vi "Check Aurora Link.vi"(0 "niUsrpRio Session":T2={"FPGA Interface"=refnum, "RIO Interface Number"=0, "Data Clock Rate"=0, "FPGA Data Clock Rate"=0, "Global Settings Register Bus"=refnum, "Radio 0 Settings Register Bus"=refnum, "Radio 1 Settings Register Bus"=refnum, "Radio Settings Bus Semaphore"=refnum, "DB Queues"=[], "Characterization Data Valid?"=FALSE, "EEPROM Header"={"Checksum"=0, "Product Code"=0, "Hardware Current Version"=0, "Hardware Oldest Compatible Version"=0, "EEPROM Map Current Version"=0, "EEPROM Map Oldest Compatible Version"=0, "User Password"="", "Pointer to Factory Header"=0, "Pointer to User Header"=0, "Recommended Interval"=0, "Number of Reserved Bytes"=9, "Number of Daughterboards"=0, "Daughterboard IDs"=[], "Daughterboard Serial Numbers"=[]}, "Device Data Header"={"Checksum"=0, "Number of Channels"=0, "Number of Gain Settings"=[], "Pointer to Characterization Data"=[], "Number of Reserved Bytes"=27, "Number of Frequencies"=[]}, "EEPROM Characterization Header"={"Checksum"=0, "Date"=timestamp(0 s since 1904-01-01), "Temperature"=0.0, "Misc. Info"="", "Pointer to Device Data Header"=0, "Number of Reserved Bytes"=28}, "Characterization Data"=[], "FPGA Current Version"=0, "FPGA Oldest Compatible Version"=0, "Fixed Logic Current Version"=0, "Fixed Logic Oldest Compatible Version"=0, "FPGA Radio Settings Bus Current Version"=0, "FPGA Radio Settings Bus Oldest Compatible Version"=0, "FPGA Board Config Current Version"=0, "FPGA Board Config Oldest Compatible Version"=0, "Daughterboard Clock Rate"=0, "daughterboard configuration session handles"=[]} {"Daughterboard Clock Rate" format="%#.3pHz"; "FPGA Data Clock Rate" format="%#.3pHz"; "Data Clock Rate" format="%#.3pHz"; "Characterization Data"."Frequencies [Hz]" format="%#_6p"; "EEPROM Characterization Header"."Pointer to Device Data Header" format="%x"; "EEPROM Characterization Header"."Checksum" format="%x"; "Device Data Header"."Pointer to Characterization Data" format="%x"; "Device Data Header"."Checksum" format="%x"; "EEPROM Header"."Pointer to User Header" format="%x"; "EEPROM Header"."Pointer to Factory Header" format="%x"; "EEPROM Header"."Product Code" format="%x"; "EEPROM Header"."Checksum" format="%x"}, 11 "error in":errorcluster) -> (4 "niUsrpRio Session (out)":T2={"FPGA Interface"=refnum, "RIO Interface Number"=0, "Data Clock Rate"=0, "FPGA Data Clock Rate"=0, "Global Settings Register Bus"=refnum, "Radio 0 Settings Register Bus"=refnum, "Radio 1 Settings Register Bus"=refnum, "Radio Settings Bus Semaphore"=refnum, "DB Queues"=[], "Characterization Data Valid?"=FALSE, "EEPROM Header"={"Checksum"=0, "Product Code"=0, "Hardware Current Version"=0, "Hardware Oldest Compatible Version"=0, "EEPROM Map Current Version"=0, "EEPROM Map Oldest Compatible Version"=0, "User Password"="", "Pointer to Factory Header"=0, "Pointer to User Header"=0, "Recommended Interval"=0, "Number of Reserved Bytes"=9, "Number of Daughterboards"=0, "Daughterboard IDs"=[], "Daughterboard Serial Numbers"=[]}, "Device Data Header"={"Checksum"=0, "Number of Channels"=0, "Number of Gain Settings"=[], "Pointer to Characterization Data"=[], "Number of Reserved Bytes"=27, "Number of Frequencies"=[]}, "EEPROM Characterization Header"={"Checksum"=0, "Date"=timestamp(0 s since 1904-01-01), "Temperature"=0.0, "Misc. Info"="", "Pointer to Device Data Header"=0, "Number of Reserved Bytes"=28}, "Characterization Data"=[], "FPGA Current Version"=0, "FPGA Oldest Compatible Version"=0, "Fixed Logic Current Version"=0, "Fixed Logic Oldest Compatible Version"=0, "FPGA Radio Settings Bus Current Version"=0, "FPGA Radio Settings Bus Oldest Compatible Version"=0, "FPGA Board Config Current Version"=0, "FPGA Board Config Oldest Compatible Version"=0, "Daughterboard Clock Rate"=0, "daughterboard configuration session handles"=[]} {"Daughterboard Clock Rate" format="%#.3pHz"; "FPGA Data Clock Rate" format="%#.3pHz"; "Data Clock Rate" format="%#.3pHz"; "Characterization Data"."Frequencies [Hz]" format="%#_6p"; "EEPROM Characterization Header"."Pointer to Device Data Header" format="%x"; "EEPROM Characterization Header"."Checksum" format="%x"; "Device Data Header"."Pointer to Characterization Data" format="%x"; "Device Data Header"."Checksum" format="%x"; "EEPROM Header"."Pointer to User Header" format="%x"; "EEPROM Header"."Pointer to Factory Header" format="%x"; "EEPROM Header"."Product Code" format="%x"; "EEPROM Header"."Checksum" format="%x"}, 6 "SFP Port Debug":T1(array[cluster]), 15 "error out":errorcluster)   [LabVIEW 2016]
uses:
  <instrlib>/niUsrpRio/Config/v1/Host/Public/niUsrpRio Session.ctl
  <instrlib>/_niInstr/Register Bus/v0/Host/Public/Register Bus Session.ctl
  <instrlib>/_niInstr/Register Bus/v0/Host/Private/Session Data.ctl
  <instrlib>/niUsrpRio/Config/v1/Host/Private/DB Queue Reference.ctl
  <instrlib>/niUsrpRio/Config/v1/Host/Private/Daughterboard Data.ctl
  <instrlib>/niUsrpRio/Config/v1/Host/Private/ATR state data.ctl
  <instrlib>/niUsrpRio/Config/v1/Host/Private/Antenna Configuration.ctl
  <instrlib>/niUsrpRio/Config/v1/Host/Private/CPLD Power Mode.ctl
  <instrlib>/niUsrpRio/Config/v1/Host/Public/EEPROM Header.ctl
  <instrlib>/niUsrpRio/Config/v1/Host/Public/EEPROM Device Data Header.ctl
  <instrlib>/niUsrpRio/Config/v1/Host/Public/EEPROM Characterization Header.ctl
  <instrlib>/niUsrpRio/Config/v1/Host/Public/Characterization Data.ctl
  <instrlib>/niUsrpRio/Config/v1/Host/Public/IQ Imbalance.ctl
  Aurora FPGA Ref.ctl
  <vilib>/rvi/errors/niLvFpgaAdjustHostInterfaceError.vi
  <vilib>/rvi/interface/nirviReadWriteControl/nirviReadWriteControl.xnode
  <vilib>/rvi/interface/Simulation/niFpgaSimulationCallBeginRW.vi
  NiFpgaLv.dll
  <instrlib>/_niInstr/Register Bus/v0/Host/niInstr Register Bus v0 Host.lvlib
  <instrlib>/niUsrpRio/Config/v1/Host/niUsrpRio Config v1 Host.lvlib
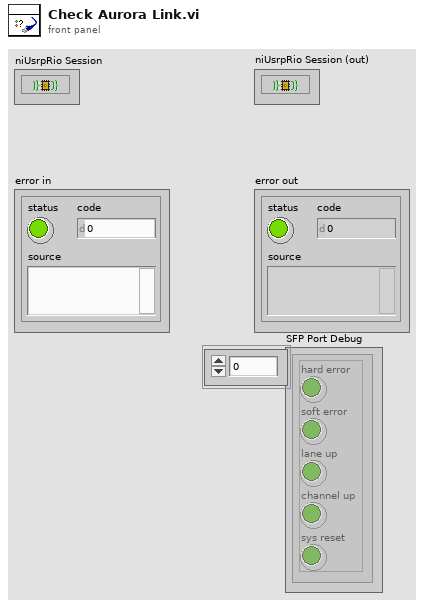
[diagram p1: front panel]
types:
  T1 = cluster{"hard error":bool, "soft error":bool, "lane up":bool, "channel up":bool, "sys reset":bool}[]
  T2 = typedef "niUsrpRio Config v1 Host.lvlib/niUsrpRio Session.ctl" = cluster{"FPGA Interface":refnum<k20>, "RIO Interface Number":u32, "Data Clock Rate":u32, "FPGA Data Clock Rate":u32, "Global Settings Register Bus":T3, "Radio 0 Settings Register Bus":T3, "Radio 1 Settings Register Bus":T3, "Radio Settings Bus Semaphore":T4, "DB Queues":T5[], "Characterization Data Valid?":bool, "EEPROM Header":T6, "Device Data Header":T7, "EEPROM Characterization Header":T8, "Characterization Data":T9[], "FPGA Current Version":u32, "FPGA Oldest Compatible Version":u32, "Fixed Logic Current Version":u32, "Fixed Logic Oldest Compatible Version":u32, "FPGA Radio Settings Bus Current Version":u32, "FPGA Radio Settings Bus Oldest Compatible Version":u32, "FPGA Board Config Current Version":u32, "FPGA Board Config Oldest Compatible Version":u32, "Daughterboard Clock Rate":u32, "daughterboard configuration session handles":u64[]}
  T3 = typedef "niInstr Register Bus v0 Host.lvlib/Register Bus Session.ctl" = refnum<queue>
  T4 = typedef "Semaphore RefNum" = refnum<k1>
  T5 = typedef "niUsrpRio Config v1 Host.lvlib/DB Queue Reference.ctl" = refnum<queue>
  T6 = typedef "niUsrpRio Config v1 Host.lvlib/EEPROM Header.ctl" = cluster{"Checksum":u32, "Product Code":u16, "Hardware Current Version":u16, "Hardware Oldest Compatible Version":u16, "EEPROM Map Current Version":u16, "EEPROM Map Oldest Compatible Version":u16, "User Password":string, "Pointer to Factory Header":u32, "Pointer to User Header":u32, "Recommended Interval":u16, "Number of Reserved Bytes":i32, "Number of Daughterboards":u8, "Daughterboard IDs":u16[], "Daughterboard Serial Numbers":string[]}
  T7 = typedef "niUsrpRio Config v1 Host.lvlib/EEPROM Device Data Header.ctl" = cluster{"Checksum":u32, "Number of Channels":u8, "Number of Gain Settings":u16[], "Pointer to Characterization Data":u32[], "Number of Reserved Bytes":i32, "Number of Frequencies":u16[]}
  T8 = typedef "niUsrpRio Config v1 Host.lvlib/EEPROM Characterization Header.ctl" = cluster{"Checksum":u32, "Date":timestamp, "Temperature":sgl, "Misc. Info":string, "Pointer to Device Data Header":u32, "Number of Reserved Bytes":i32}
  T9 = typedef "niUsrpRio Config v1 Host.lvlib/Characterization Data.ctl" = cluster{"Gains[dB]":dbl[], "Frequencies [Hz]":dbl[], "IQ Imbalance Table":T10[], "Measured Gains[dB]":dbl[][]}
  T10 = typedef "niUsrpRio Config v1 Host.lvlib/IQ Imbalance.ctl" = cluster{"Gain Imbalance [linear]":dbl, "Phase Imbalance [radians]":dbl, "Offset":cdb}
  T11 = typedef "Aurora FPGA Ref.ctl" = refnum<k20>
  T12 = cluster{"hard error":bool, "soft error":bool, "lane up":bool, "channel up":bool, "sys reset":bool}
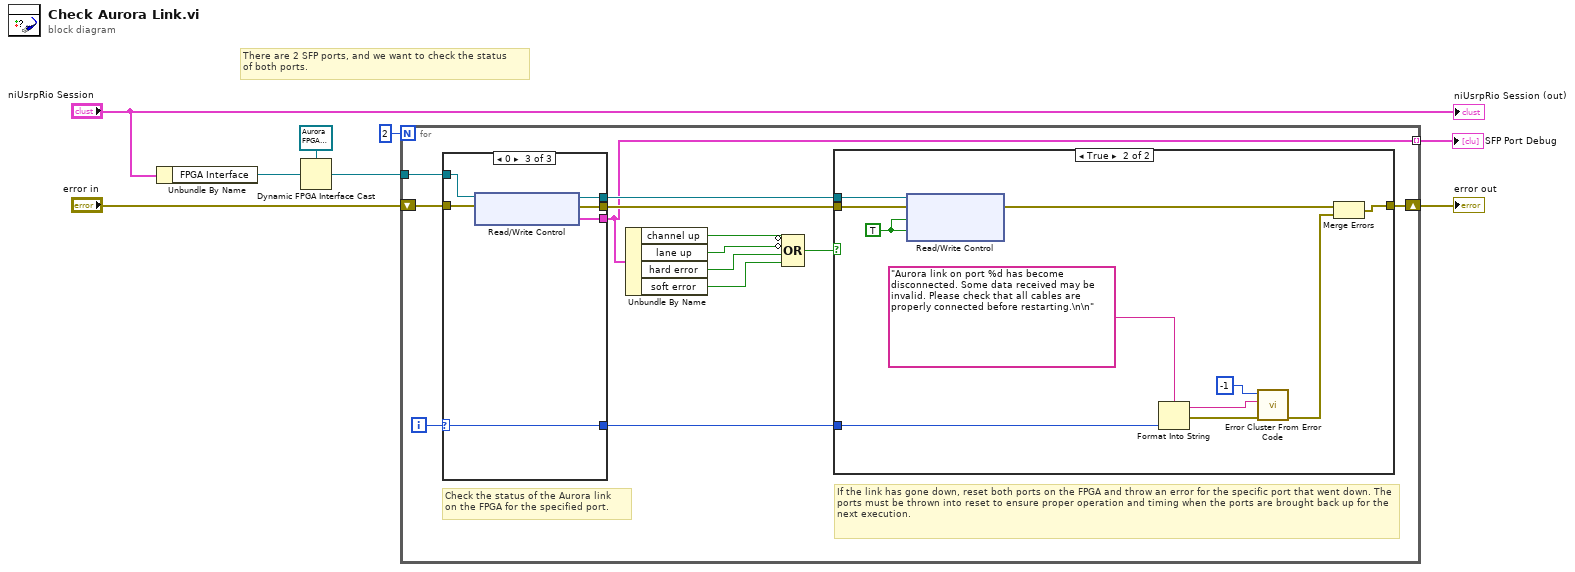
[diagram p0: block diagram]
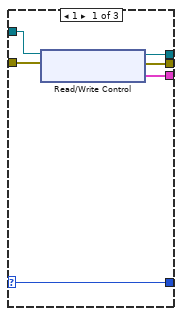
[diagram p3: hidden frame]
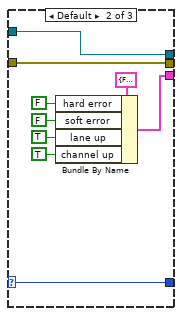
[diagram p4: hidden frame]
diagram:
  # "There are 2 SFP ports, and we want to check the status\nof both ports."
  n1 = Unbundle By Name("niUsrpRio Session") -> ("FPGA Interface"=w8:refnum<k20>)
  n2 = Dynamic FPGA Interface Cast(Session In=T11 refnum ("USRP RIO Streaming Xcvr FPGA VI Reference"), Type=w8) -> (Session Out=w6:T11)
  n3 = for {
    N: 2 -> [_]
    tunnel: w6 -> [w21]
    shift-right: [w17] -> w4
    shift-left: "error in" -> [w20]
    tunnel: [w9] -> w1 mode=indexing
    i -> [w15]
    # "If the link has gone down, reset both ports on the FPGA and throw an error for the specific port that went down. The ports must be thrown into reset to ensure proper operation and timing when the ports are brought back up for the next execution."
    # "Check the status of the Aurora link \non the FPGA for the specified port."
    n4 = case shown="0" w15 {
      selector: w15 -> [w34 w46 w49]
      tunnel: w21 -> [w39 w47 w54]
      tunnel: [w38 w44 w53] -> w9
      tunnel: w20 -> [w37 w48 w52]
      tunnel: [w36 w48 w51] -> w19
      tunnel: [w35 w47 w50] -> w18
      tunnel: [w34 w46 w49] -> w16
      frame 1 {
        n5 = xnode "Read/Write Control"("FPGA VI Reference In"=w39, "error in"=w37) -> ("FPGA VI Reference Out"=w35:T11, "error out"=w36:errorcluster, "sfp 1.debug info"=w38:T12)
      }
      frame Default {
        n6 = Bundle By Name(cluster=T12 {"hard error"=FALSE, "soft error"=FALSE, "lane up"=FALSE, "channel up"=FALSE, "sys reset"=FALSE} ("sfp 0.debug info"), "hard error"=FALSE, "soft error"=FALSE, "lane up"=TRUE, "channel up"=TRUE) -> (w44:T12)
      }
      frame 0 {
        n7 = xnode "Read/Write Control"("FPGA VI Reference In"=w54, "error in"=w52) -> ("FPGA VI Reference Out"=w50:T11, "error out"=w51:errorcluster, "sfp 0.debug info"=w53:T12)
      }
    }
    n8 = Unbundle By Name(w9) -> ("channel up"=w14:bool, "lane up"=w12:bool, "hard error"=w11:bool, "soft error"=w10:bool)
    n9 = Compound Arithmetic op=OR(invert w14, invert w12, w11, w10) -> (w13:bool)
    n10 = case shown="True" w13 {
      tunnel: w19 -> [w22 w32]
      tunnel: w18 -> [_ w33]
      tunnel: [w22 w30] -> w17
      tunnel: w16 -> [_ w26]
      frame False {
      }
      frame True {
        w31 = TRUE
        n11 = xnode "Read/Write Control"("FPGA VI Reference In"=w33, "error in"=w32, "sfp 0.core reset"=w31, "sfp 1.core reset"=w31) -> ("error out"=w23:errorcluster)  [unwired: 1 out]
        n12 = Format Into String(format string="Aurora link on port %d has become disconnected. Some data received may be invalid. Please check that all cables are properly connected before restarting.\n\n" ("error message (\"\")"), w26) -> (resulting string=w27:string, error out=w28:errorcluster)  [unwired: 2 in]
        n13 = call <vilib>:"Error Cluster From Error Code.vi"("error in (no error)"=w28, "error message (\"\")"=w27, "error code (0)"=-1) -> ("error out"=w24:errorcluster)  [unwired: 6 in]
        n14 = Merge Errors(w23, w24) -> (w30:errorcluster)
      }
    }
  }
  "error out" <- w4
  "SFP Port Debug" <- w1
  "niUsrpRio Session (out)" <- "niUsrpRio Session"
